vi "工具_索引变量属性-temp.vi"(1 "模块名称":string) -> (0 "数据属性数组":T1(array[cluster]))   [LabVIEW 2014]
doc: "该模板用于创建子VI。"
uses:
  glb/glb_data.vi
panel:
  out "error out":errorcluster caption="错误输出"
  in  "error in (no error)":errorcluster caption="错误输入（无错误）"
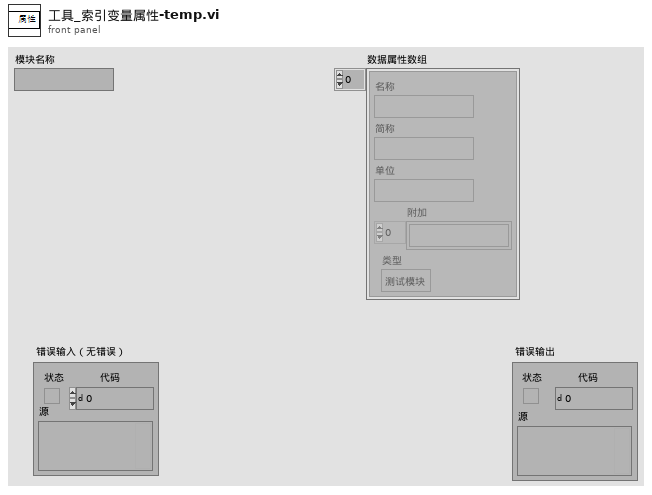
[diagram p1: front panel]
types:
  T1 = cluster{"名称":string, "简称":string, "单位":string, "附加":string[], "类型":enum16{"测试模块", "FPGA", "cRIO", "其他设备", "总体展示"}}[]
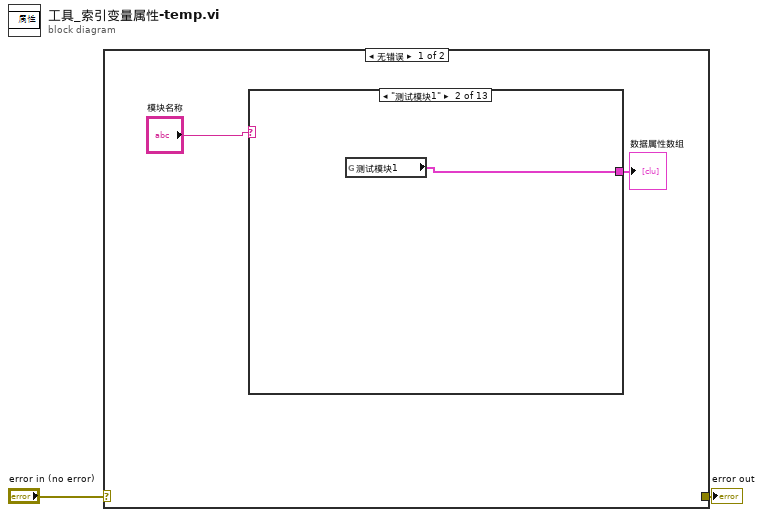
[diagram p0: block diagram]
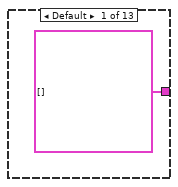
[diagram p2: hidden frame]
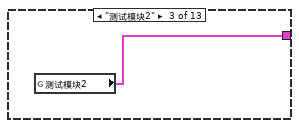
[diagram p3: hidden frame]
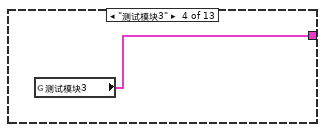
[diagram p4: hidden frame]
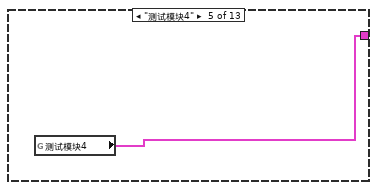
[diagram p5: hidden frame]
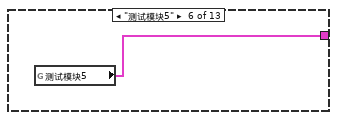
[diagram p6: hidden frame]
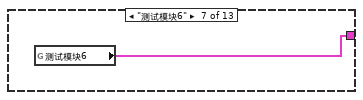
[diagram p7: hidden frame]
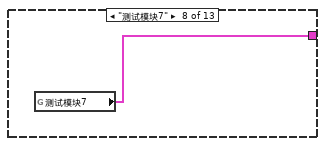
[diagram p8: hidden frame]
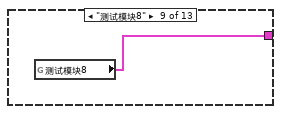
[diagram p9: hidden frame]
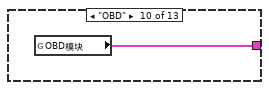
[diagram p10: hidden frame]
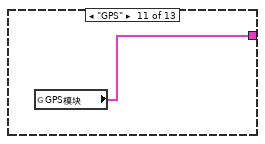
[diagram p11: hidden frame]
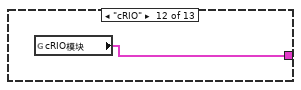
[diagram p12: hidden frame]
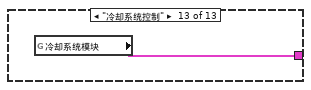
[diagram p13: hidden frame]
diagram:
  n1 = case shown="无错误" "error in (no error)" {
    selector: "error in (no error)" -> [_ w18]
    tunnel: [_ w18] -> w1
    frame No Error {
      n2 = case shown="\"测试模块1\"" "模块名称" {
        tunnel: [T1 [] ("cRIO模块") w6 w7 w8 w9 w10 w11 w12 w13 w14 w15 w16 w17] -> w3
        frame Default {
        }
        frame "测试模块1" {
          n3 = global read "配置变量_temp.vi" "测试模块1"() -> (w6:T1)
        }
        frame "测试模块2" {
          n4 = global read "配置变量_temp.vi" "测试模块2"() -> (w7:T1)
        }
        frame "测试模块3" {
          n5 = global read "配置变量_temp.vi" "测试模块3"() -> (w8:T1)
        }
        frame "测试模块4" {
          n6 = global read "配置变量_temp.vi" "测试模块4"() -> (w9:T1)
        }
        frame "测试模块5" {
          n7 = global read "配置变量_temp.vi" "测试模块5"() -> (w10:T1)
        }
        frame "测试模块6" {
          n8 = global read "配置变量_temp.vi" "测试模块6"() -> (w11:T1)
        }
        frame "测试模块7" {
          n9 = global read "配置变量_temp.vi" "测试模块7"() -> (w12:T1)
        }
        frame "测试模块8" {
          n10 = global read "配置变量_temp.vi" "测试模块8"() -> (w13:T1)
        }
        frame "OBD" {
          n11 = global read "glb_data.vi" "OBD模块"() -> (w14:T1)
        }
        frame "GPS" {
          n12 = global read "glb_data.vi" "GPS模块"() -> (w15:T1)
        }
        frame "cRIO" {
          n13 = global read "glb_data.vi" "cRIO模块"() -> (w16:T1)
        }
        frame "冷却系统控制" {
          n14 = global read "glb_data.vi" "冷却系统模块"() -> (w17:T1)
        }
      }
      "数据属性数组" <- w3
    }
    frame Error {
    }
  }
  "error out" <- w1
